vi "tvac_gui_chamber.vi"() -> ()   [LabVIEW 2016]
uses:
  <vilib>/httpClient/LabVIEWHTTPClient.lvlib
  <vilib>/httpClient/ClientHandle.ctl
  msg7171_linux.llb/send single message.vi
  <vilib>/httpClient/POSTBuffer.vi
panel:
  out "array w/ subset deleted":waveform(dbl)[](array[waveform])
  in  "AlarmColor":u32(colorbox)
  in  "Alarm String":string
  in  "Plot Color":u32(colorbox)=16860
  in  "Temperature":dbl format="%#_13g"
  in  "TC Label":string
  in  "Graph ON/OFF":u32(colorbox)=4250624
  in  "index (col)":i32
  in  "index (row)":i32
  out "working array":bool[](array[boolean])
  in  "Local Debug":bool
  in  "Tab Control":enum32{"TCs"}(tab)
  in  "Graphing Selection":u16(ring) items=["User Selection", "Graph All Thermocouples", "Clear Graph"]
  in  "Time Scale":u16(ring) items=["Minutes", "Hours", "Seconds"]
  out "Waveform Chart":waveform(dbl)[](graph)
  out "Thermocouples":T1(array[cluster])
  in  "exit":bool
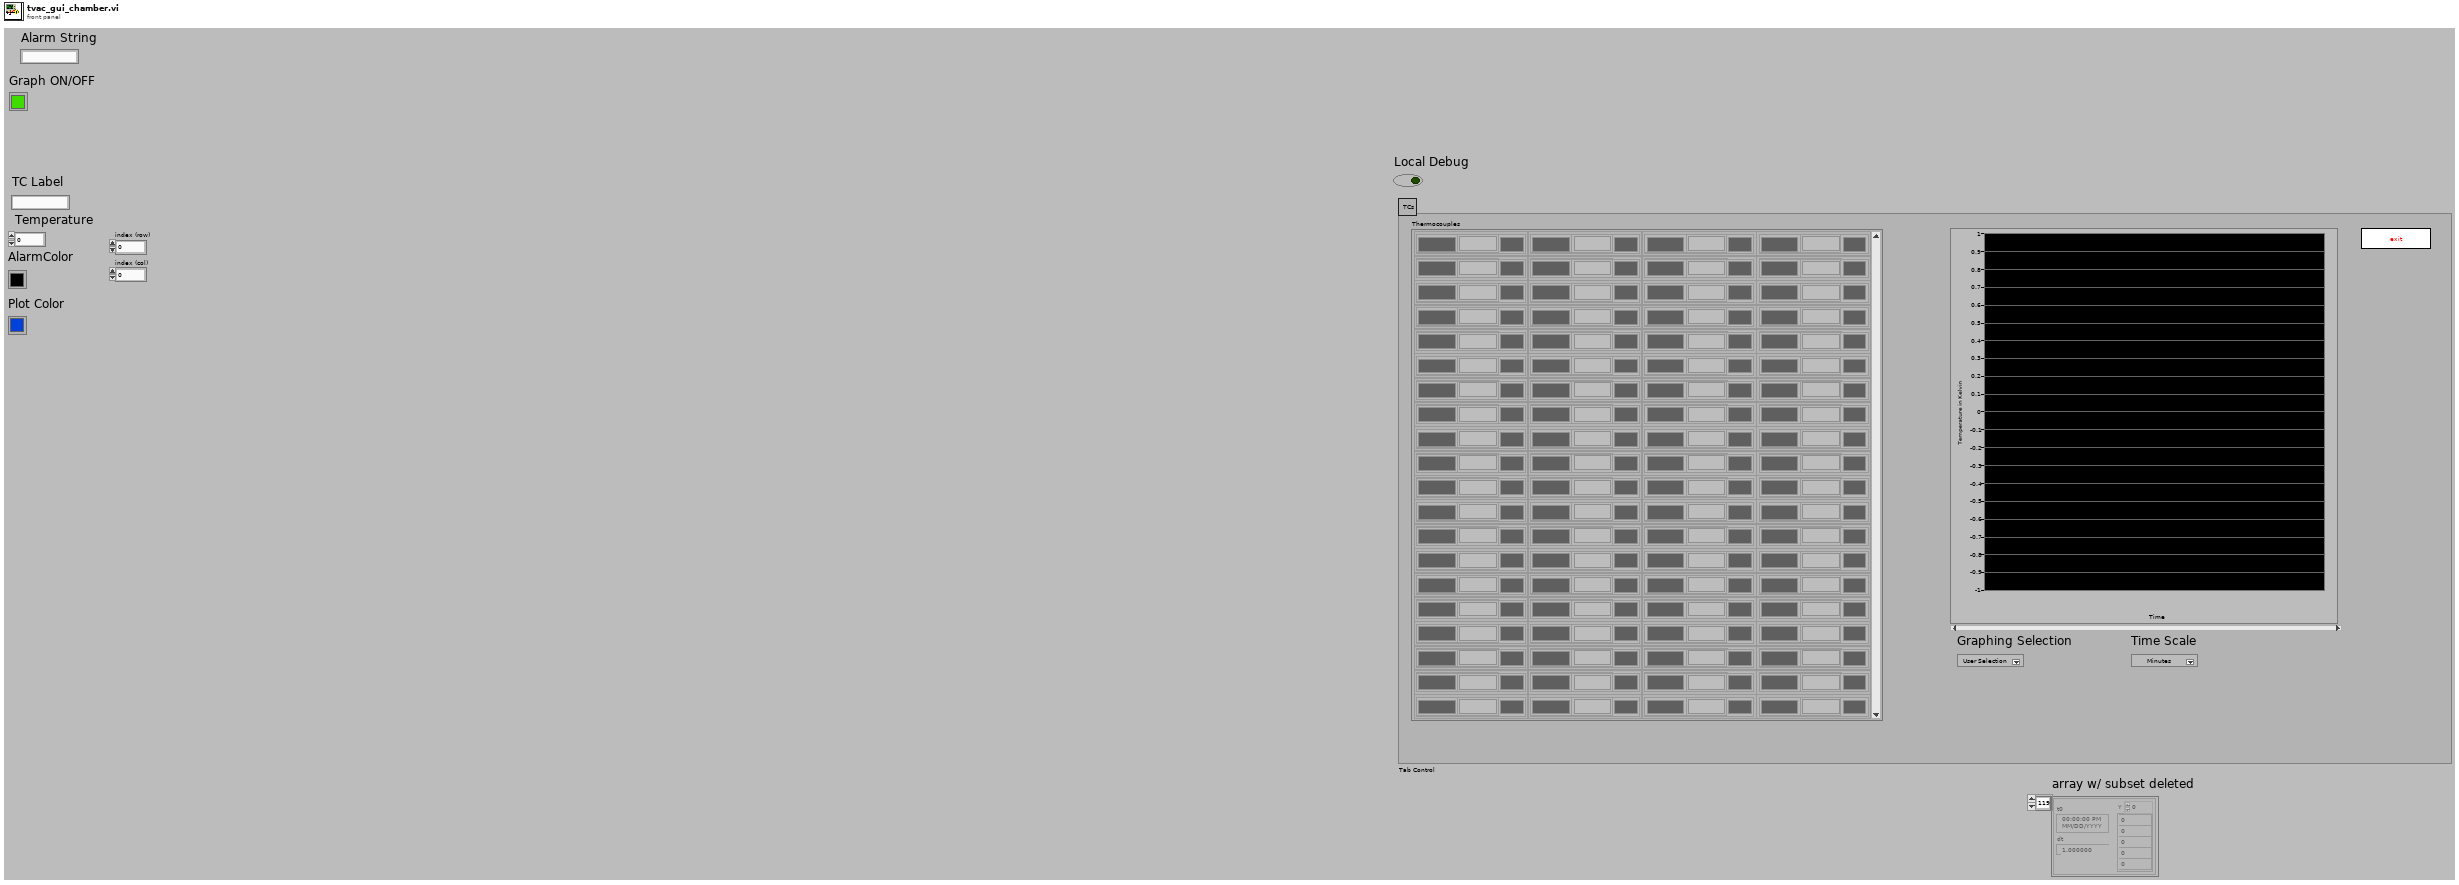
[diagram p1: front panel]
types:
  T1 = cluster{"TC Label":string, "Alarm Status":string, "Alarm Color":u32, "Temperature":string, "PlotColor":u32, "Graph On/Off":u32}[][]
  T2 = typedef "LabVIEWHTTPClient.lvlib/ClientHandle.ctl" = refnum<k1>
  T3 = cluster{"go":bool, "Http session":T2, "URL prefex":string, "index (row)":i32, "index (col)":i32, "Graph ON/OFF":u32, "TC Label":string, "Temperature":dbl, "AlarmColor":u32, "Plot Color":u32, "Alarm String":string, "Thermocouples":cluster{"TC Label":string, "Alarm Status":string, "Alarm Color":u32, "Temperature":string, "PlotColor":u32, "Graph On/Off":u32}[][], "working array":bool[], "i":i32, "NumberTCs":i32, "Waveform Chart":waveform(dbl)[]}
  T4 = cluster{"TC Label":string, "Alarm Status":string, "Alarm Color":u32, "Temperature":string, "PlotColor":u32, "Graph On/Off":u32}
  T5 = typedef "LVPoint32TypeDef.ctl" = cluster{"Horizontal":i32, "Vertical":i32}
  T6 = typedef "LVPositionTypeDef.ctl" = cluster{"Left":i32, "Top":i32}
  T7 = typedef "LVRangeTypeDef.ctl" = cluster{"Minimum":dbl, "Maximum":dbl, "Increment":dbl, "Minor Increment":dbl, "Start":dbl}
  T8 = cluster{"time":string, "TCs":cluster{"thermocouple":i32, "time":dbl, "temp":dbl, "working":bool, "alarm":i32}[]}
  T9 = cluster{"thermocouple":i32, "time":dbl, "temp":dbl, "working":bool, "alarm":i32}[]
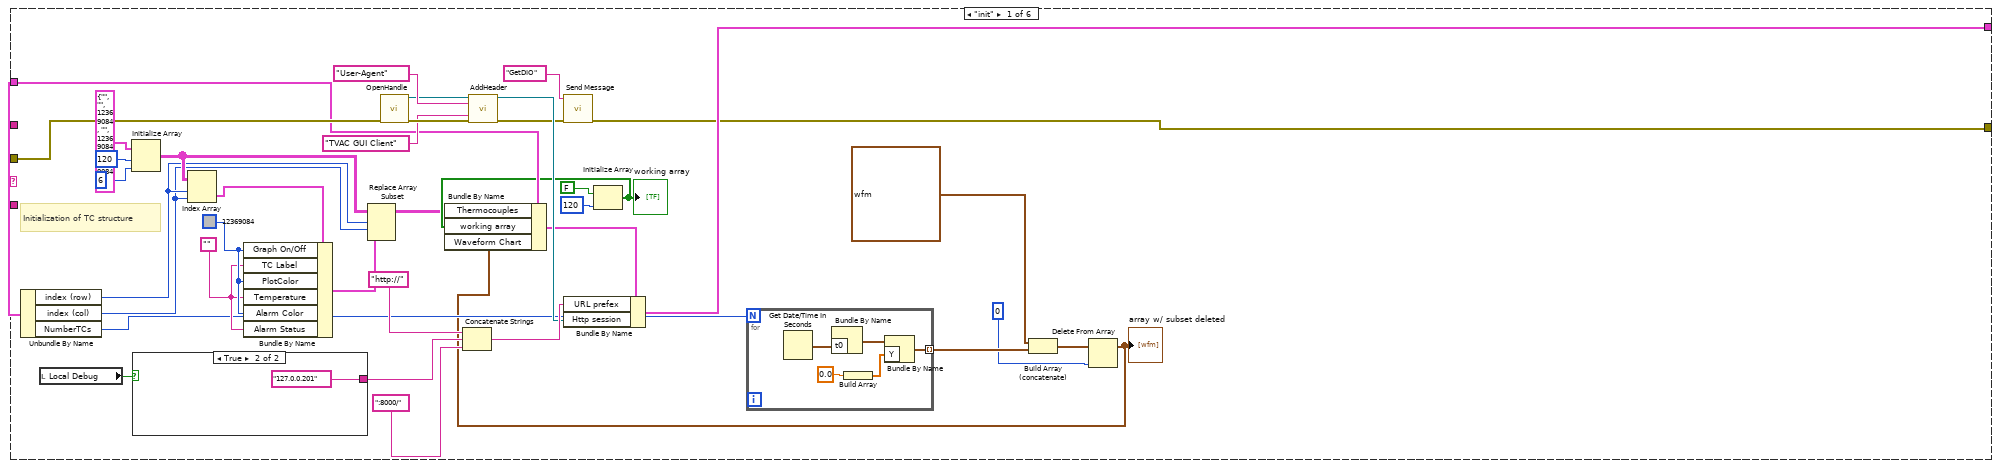
[diagram p2: hidden frame]
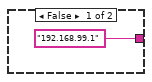
[diagram p3: hidden frame]
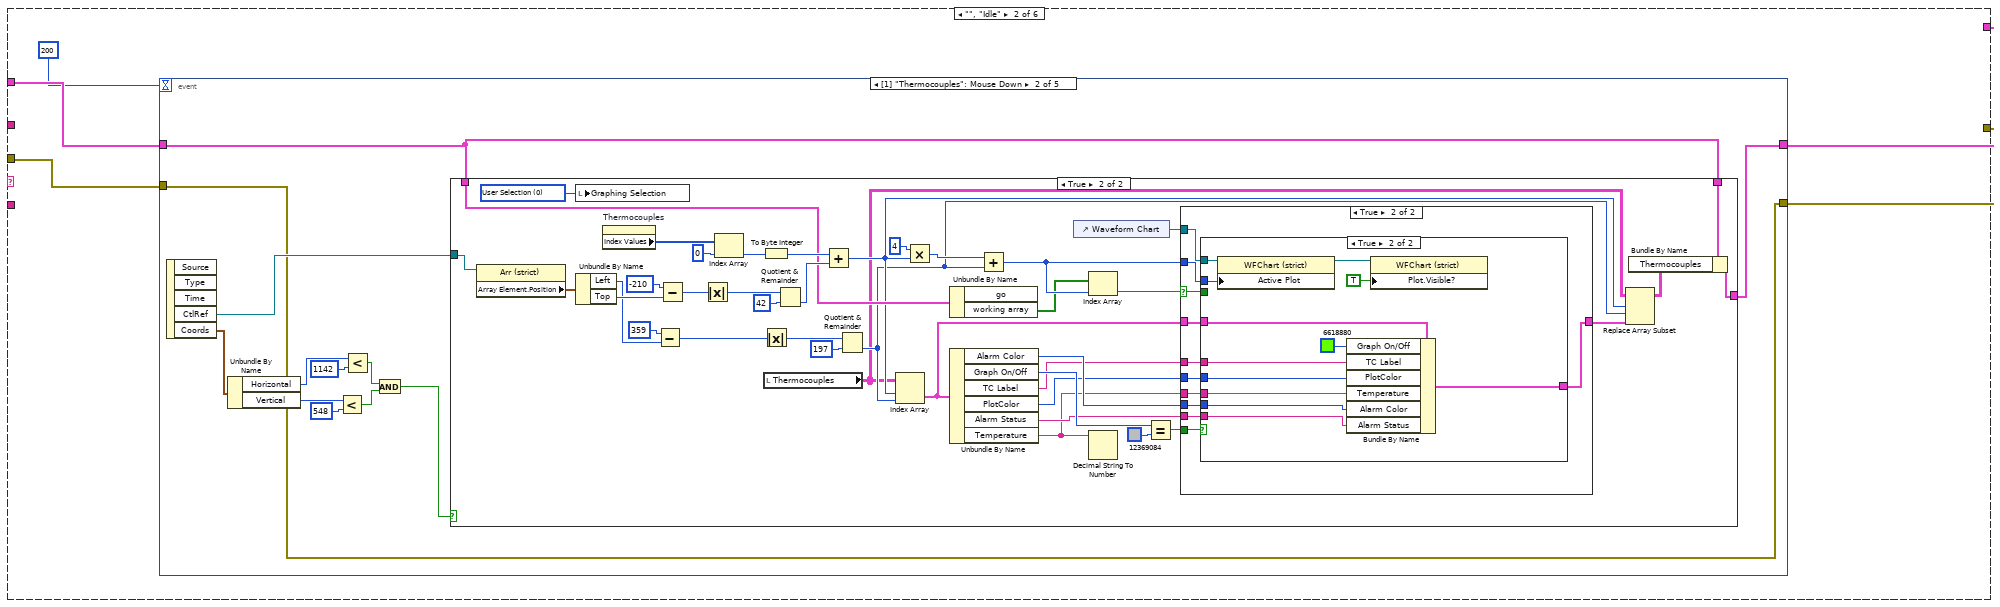
[diagram p4: hidden frame]
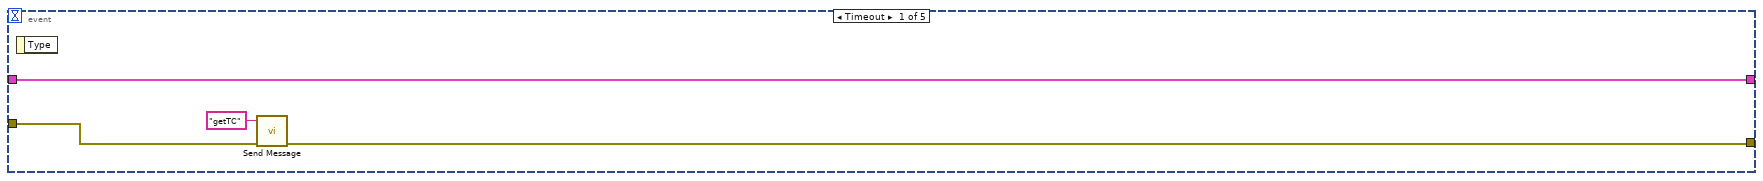
[diagram p5: hidden frame]
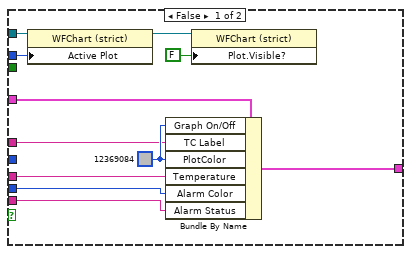
[diagram p8: hidden frame]
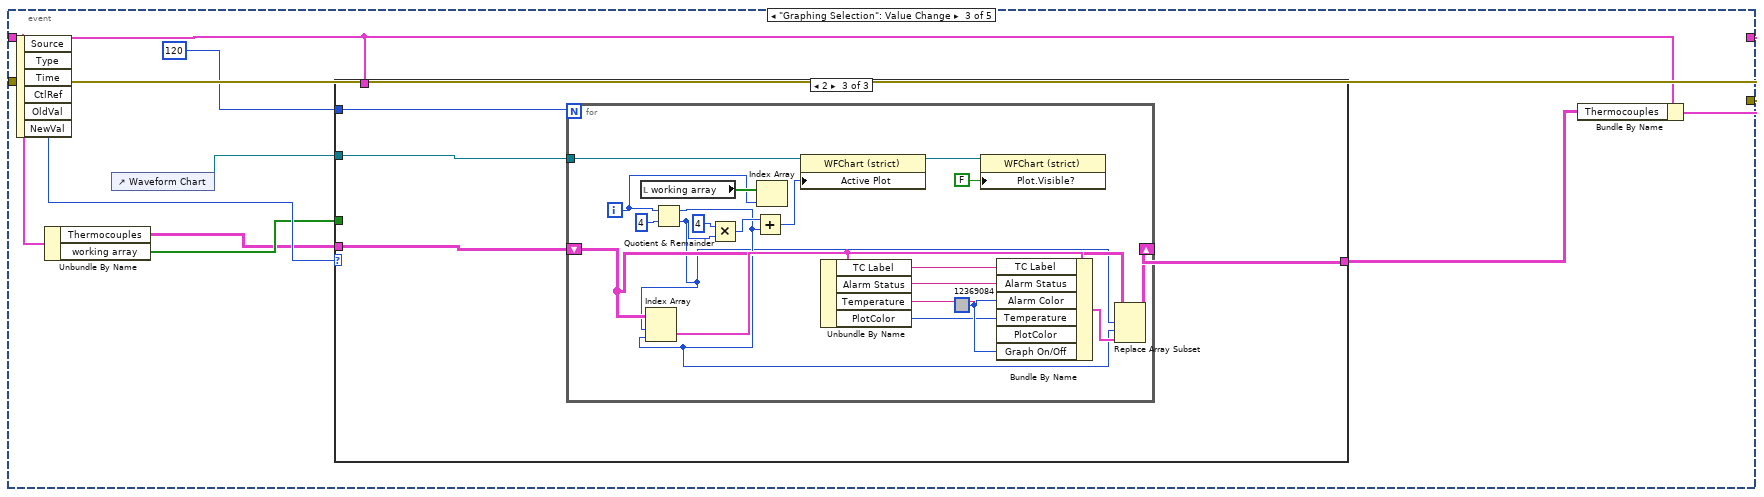
[diagram p9: hidden frame]
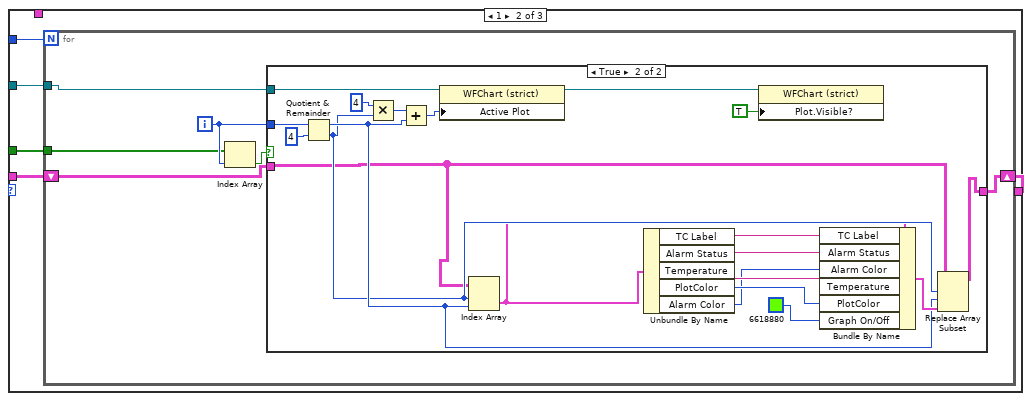
[diagram p11: hidden frame]
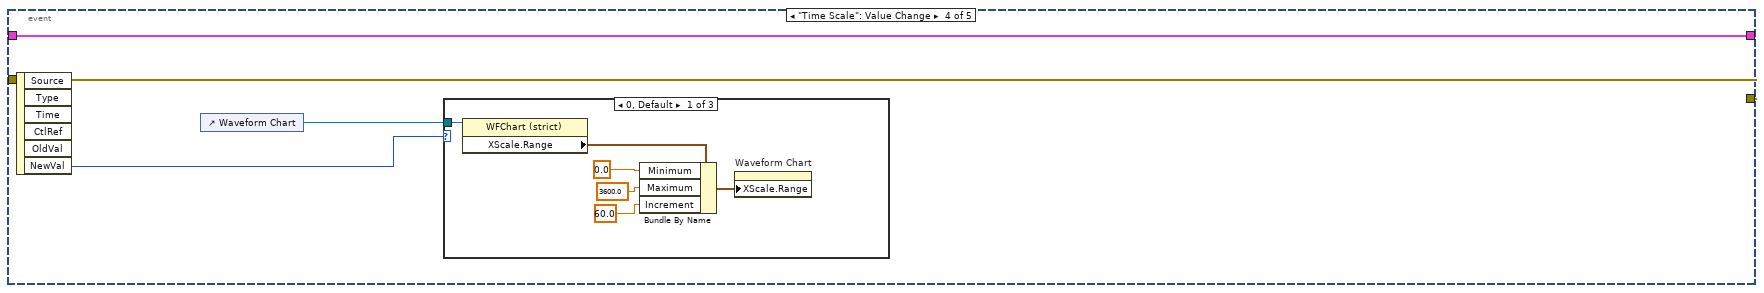
[diagram p13: hidden frame]
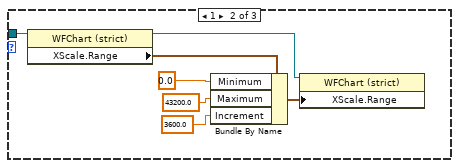
[diagram p14: hidden frame]
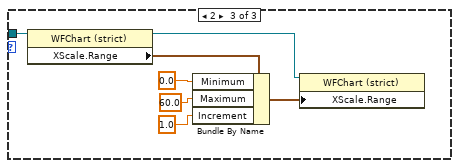
[diagram p15: hidden frame]
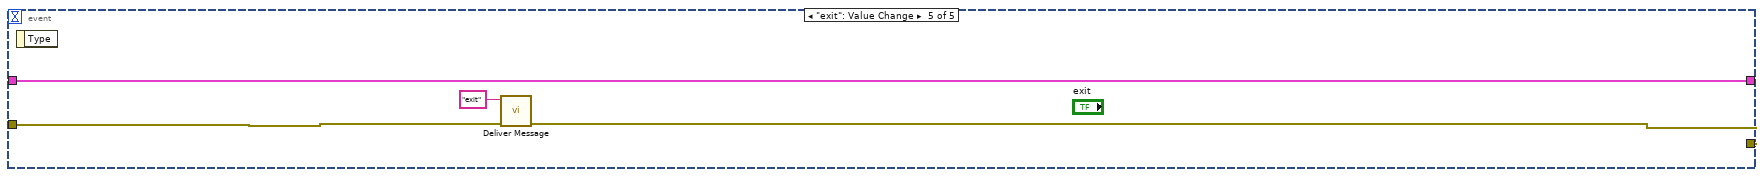
[diagram p16: hidden frame]
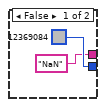
[diagram p17: hidden frame]
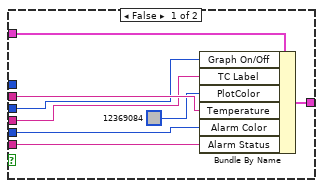
[diagram p18: hidden frame]
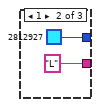
[diagram p19: hidden frame]
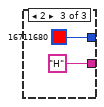
[diagram p20: hidden frame]
diagram:
  w19 = ""  # URL prefex
  w20 = T2 refnum  # Http session
  w21 = TRUE  # go
  n1 = call "Register Module.vi"() -> ("error out"=w17:errorcluster)  [unwired: 10 in, 1 out]
  n2 = call-poly "Send Message.vi"("error in (no error)"=w17, "event"="init") -> ("error out"=w16:errorcluster)  [unwired: 9 in]
  n3 = local read "Waveform Chart"() -> (w3:waveform(dbl)[])
  n4 = local read "Thermocouples"() -> (w2:T1)
  n5 = Bundle("go"=w21, "Http session"=w20, "URL prefex"=w19, "index (row)"="index (row)", "index (col)"="index (col)", "Graph ON/OFF"="Graph ON/OFF", "TC Label"="TC Label", "Temperature"="Temperature", "AlarmColor"="AlarmColor", "Plot Color"="Plot Color", "Alarm String"="Alarm String", "Thermocouples"=w2, "working array"=bool[] [TRUE, TRUE, TRUE, TRUE, TRUE, TRUE, TRUE, TRUE, TRUE, TRUE, TRUE, TRUE, TRUE, TRUE, TRUE, TRUE, TRUE, TRUE, TRUE, TRUE, TRUE, TRUE, TRUE, TRUE, TRUE, TRUE, TRUE, TRUE, TRUE, TRUE, TRUE, TRUE, TRUE, TRUE, TRUE, TRUE, TRUE, TRUE, TRUE, TRUE, TRUE, TRUE, TRUE, TRUE, TRUE, TRUE, TRUE, TRUE, TRUE, TRUE, TRUE, TRUE, TRUE, TRUE, TRUE, TRUE, TRUE, TRUE, TRUE, TRUE, TRUE, TRUE, TRUE, TRUE, TRUE, TRUE, TRUE, TRUE, TRUE, TRUE, TRUE, TRUE, TRUE, TRUE, TRUE, TRUE, TRUE, TRUE, TRUE, TRUE, TRUE, TRUE, TRUE, TRUE, TRUE, TRUE, TRUE, TRUE, TRUE, TRUE, TRUE, TRUE, TRUE, TRUE, TRUE, TRUE, TRUE, TRUE, TRUE, TRUE, TRUE, TRUE, TRUE, TRUE, TRUE, TRUE, TRUE, TRUE, TRUE, TRUE, TRUE, TRUE, TRUE, TRUE, TRUE, TRUE, TRUE, TRUE, TRUE, TRUE], "i"=0, "NumberTCs"=120, "Waveform Chart"=w3) -> (w7:T3)  [unwired: 1 in]
  n6 = while {
    shift-left: w7 -> [w26]
    shift-right: [w23] -> _
    shift-right: [w24] -> w1
    shift-left: w16 -> [w31]
    stop <- w22 continue-if-true
    n7 = call "Get Message.vi"("error in (no error)"=w31) -> ("error out"=w29:errorcluster, "event buffer"=w30:string, "event"=w28:string, "source"=w27:string)  [unwired: 7 in]
    n8 = case shown="\"getTC\"" w28 {
      selector: w28 -> [_ _ _ _ _ w432]
      tunnel: [w61 w78 w269 w401 w430 w434] -> w23
      tunnel: w26 -> [w41 w80 w275 w402 w425 w434]
      tunnel: w30 -> [_ _ _ _ _ _]
      tunnel: w29 -> [w64 w79 w296 w404 w428 w433]
      tunnel: [w57 w77 w270 w404 w427 w431] -> w25
      tunnel: w27 -> [_ _ _ _ _ _]
      frame "init" {
        w46 = ""
        w47 = u32 12369084 ("PlotColor")
        # "Initialization of TC structure"
        n9 = Unbundle By Name(w41) -> ("index (row)"=w49:i32, "index (col)"=w48:i32, "NumberTCs"=w38:i32)
        n10 = local read "Local Debug"() -> (w54:bool)
        n11 = Initialize Array(T4 {"TC Label"="", "Alarm Status"="", "Alarm Color"=12369084, "Temperature"="", "PlotColor"=12369084, "Graph On/Off"=12369084}, 120 ("dimension size"), 6 ("dimension size")) -> (w50:T1)
        n12 = case shown="True" w54 {
          tunnel: ["192.168.99.1" ("Address") "127.0.0.201" ("Address")] -> w55
          frame False {
          }
          frame True {
          }
        }
        n13 = Index Array(array=w50, index (row)=w49, index (col)=w48) -> (element=w45:T4)
        n14 = Bundle By Name(cluster=w45, "Graph On/Off"=w47, "TC Label"=w46, "PlotColor"=w47, "Temperature"=w46, "Alarm Color"=w47, "Alarm Status"=w46) -> (w44:T4)
        n15 = Replace Array Subset(array=w50, new element=w44, index (row)=w49, index (col)=w48) -> (w32:T1)
        n16 = call <vilib>:"OpenHandle.vi"("error in (no error)"=w64) -> ("client handle out"=w65:T2, "error out"=w68:errorcluster)  [unwired: 13 in]
        n17 = Concatenate Strings("http://" ("url"), w55, ":8000/" ("url")) -> (w60:string)
        n18 = call <vilib>:"AddHeader.vi"("client handle"=w65, "header"="User-Agent", "value"="TVAC GUI Client", "error in (no error)"=w68) -> ("client handle out"=w59:T2, "error out"=w58:errorcluster)  [unwired: 10 in]
        n19 = call-poly "Send Message.vi"("error in (no error)"=w58, "event"="GetDIO") -> ("error out"=w57:errorcluster)  [unwired: 9 in]
        n20 = Initialize Array(FALSE ("Boolean"), 120 ("dimension size")) -> (w39:bool[])
        "working array" <- w39
        n21 = for {
          N: w38 -> [_]
          tunnel: [w69] -> w36 mode=indexing
          n22 = Get Date/Time In Seconds() -> (seconds since 1Jan1904=w73:timestamp)
          n23 = Bundle By Name("t0"=w73) -> (w70:waveform(dbl))  [unwired: 1 in]
          n24 = Build Array(0.0) -> (w72:dbl[])
          n25 = Bundle By Name(cluster=w70, "Y"=w72) -> (w69:waveform(dbl))
        }
        n26 = Build Array (concatenate)(waveform(dbl) {"t0"=timestamp(0 s since 1904-01-01), "dt"=1.0, "Y"=[0.0]} ("element"), w36) -> (w37:waveform(dbl)[])
        n27 = Delete From Array(array=w37, index=0) -> (array with subset deleted=w35:waveform(dbl)[])  [unwired: 1 in, 1 out]
        "array w/ subset deleted" <- w35
        n28 = Bundle By Name(cluster=w41, "Thermocouples"=w32, "working array"=w39, "Waveform Chart"=w35) -> (w40:T3)
        n29 = Bundle By Name(cluster=w40, "URL prefex"=w60, "Http session"=w59) -> (w61:T3)
      }
      frame "", "Idle" {
        n30 = event shown="[1] \"Thermocouples\": Mouse Down" {
          selector: _ -> [_ _ _ _ _]
          dyn-events: _ -> [_ _ _ _ _]
          timeout: 200 ("milliseconds to wait") -> [_ _ _ _ _]
          tunnel: w79 -> [w82 w85 w180 w241 w266]
          tunnel: [w81 w85 w180 w241 w264] -> w77
          tunnel: [w84 w86 w175 w242 w267] -> w78
          tunnel: w80 -> [w84 w87 w176 w242 w267]
          event Timeout {
            n31 = event-data() -> ()  [unwired: 1 in, 1 out]
            n32 = call-poly "Send Message.vi"("error in (no error)"=w82, "event"="getTC") -> ("error out"=w81:errorcluster)  [unwired: 9 in]
          }
          event "Thermocouples": Mouse Down {
            n33 = event-data() -> ("CtlRef"=w89:refnum<vi>, "Coords"=w96:T5)  [unwired: 1 in, 3 out]
            n34 = Unbundle By Name(w96) -> ("Horizontal"=w94:i32, "Vertical"=w91:i32)
            n35 = Less?(x=w91, y=548) -> (x < y?=w90:bool)
            n36 = Less?(x=w94, y=1142) -> (x < y?=w95:bool)
            n37 = And(x=w95, y=w90) -> (x .and. y?=w88:bool)
            n38 = case shown="True" w88 {
              tunnel: w89 -> [_ w138]
              tunnel: w87 -> [_ w108]
              tunnel: w87 -> [w97 w106]
              tunnel: [w97 w98] -> w86
              frame False {
              }
              frame True {
                w132 = u16 0 items=["User Selection", "Graph All Thermocouples", "Clear Graph"] ("Graphing Selection")
                n39 = property class="Arr (strict)"(reference=w138) -> ("Array Element.Position"=w130:T6)  [unwired: 1 in, 2 out]
                n40 = local write "Graphing Selection"(w132) -> ()
                n41 = Unbundle By Name(w130) -> ("Left"=w127:i32, "Top"=w131:i32)
                n42 = property on="Thermocouples" class="Arr (strict)"() -> ("Index Values"=w121:u32[])  [unwired: 2 in, 2 out]
                n43 = Subtract(x=359, y=w127) -> (x-y=w126:i32)
                n44 = Subtract(x=-210, y=w131) -> (x-y=w118:i32)
                n45 = Absolute Value(x=w118) -> (abs(x)=w129:i32)
                n46 = Index Array(array=w121, index=0) -> (element=w117:u32)
                n47 = To Byte Integer(number=w117) -> (8bit integer=w116:i8)
                n48 = Absolute Value(x=w126) -> (abs(x)=w125:i32)
                n49 = local read "Thermocouples"() -> (w99:T1)
                n50 = Quotient & Remainder(x=w129, y=42) -> (floor(x/y)=w114:i32)  [unwired: 1 out]
                n51 = Add(x=w116, y=w114) -> (x+y=w101:i32)
                n52 = Quotient & Remainder(x=w125, y=197 ("Numeric 2")) -> (floor(x/y)=w100:i32)  [unwired: 1 out]
                n53 = Index Array(array=w99, index (row)=w101, index (col)=w100) -> (element=w102:T4)
                n54 = Multiply(x=4, y=w101) -> (x*y=w122:i32)
                n55 = Unbundle By Name(w108) -> ("working array"=w107:bool[])  [unwired: 1 out]
                n56 = Unbundle By Name(w102) -> ("Alarm Color"=w136:u32, "Graph On/Off"=w135:u32, "TC Label"=w134:string, "PlotColor"=w113:u32, "Alarm Status"=w133:string, "Temperature"=w104:string)
                n57 = Add(x=w122, y=w100) -> (x+y=w110:i32)
                n58 = control-ref of="Waveform Chart"() -> (w137:refnum<vi>)
                n59 = Index Array(array=w107, index=w110) -> (element=w109:bool)
                n60 = Decimal String To Number(string=w104) -> ()  [unwired: 2 in, 2 out]
                n61 = Equal?(x=w135, y=u32 12369084) -> (x = y?=w111:bool)
                n62 = case shown="True" w109 {
                  selector: w109 -> [_ w144]
                  tunnel: w137 -> [_ w150]
                  tunnel: w136 -> [_ w149]
                  tunnel: w134 -> [_ w148]
                  tunnel: w133 -> [_ w147]
                  tunnel: w110 -> [_ w140]
                  tunnel: w113 -> [_ w146]
                  tunnel: w111 -> [_ w145]
                  tunnel: w104 -> [_ w143]
                  tunnel: [w139 w142] -> w103
                  tunnel: w102 -> [w139 w141]
                  frame False {
                  }
                  frame True {
                    n63 = case shown="True" w145 {
                      tunnel: w150 -> [w160 w171]
                      tunnel: w149 -> [w154 w166]
                      tunnel: w148 -> [w155 w165]
                      tunnel: w147 -> [w156 w167]
                      tunnel: w146 -> [_ w169]
                      tunnel: w144 -> [_ _]
                      tunnel: w143 -> [w157 w168]
                      tunnel: [w152 w164] -> w142
                      tunnel: w141 -> [w153 w163]
                      tunnel: w140 -> [w151 w162]
                      frame False {
                        w158 = u32 12369084
                        n64 = property on="Property Node" class="WFChart (strict)"(reference=w160, "Active Plot"=w151) -> (reference out=w161:refnum<vi>)  [unwired: 1 in, 1 out]
                        n65 = Bundle By Name(cluster=w153, "Graph On/Off"=w158, "TC Label"=w155, "PlotColor"=w158, "Temperature"=w157, "Alarm Color"=w154, "Alarm Status"=w156) -> (w152:T4)
                        n66 = property class="WFChart (strict)"(reference=w161, "Plot.Visible?"=FALSE ("Plot.Visible")) -> ()  [unwired: 1 in, 2 out]
                      }
                      frame True {
                        n67 = property class="WFChart (strict)"(reference=w171, "Active Plot"=w162) -> (reference out=w172:refnum<vi>)  [unwired: 1 in, 1 out]
                        n68 = Bundle By Name(cluster=w163, "Graph On/Off"=u32 6618880, "TC Label"=w165, "PlotColor"=w169, "Temperature"=w168, "Alarm Color"=w166, "Alarm Status"=w167) -> (w164:T4)
                        n69 = property class="WFChart (strict)"(reference=w172, "Plot.Visible?"=TRUE ("Plot.Visible")) -> ()  [unwired: 1 in, 2 out]
                      }
                    }
                  }
                }
                n70 = Replace Array Subset(array=w99, new element=w103, index (row)=w101, index (col)=w100) -> (w105:T1)
                n71 = Bundle By Name(cluster=w106, "Thermocouples"=w105) -> (w98:T3)
              }
            }
          }
          event "Graphing Selection": Value Change {
            n72 = event-data() -> ("NewVal"=w181:u16)  [unwired: 1 in, 5 out]
            n73 = Unbundle By Name(w176) -> ("Thermocouples"=w174:T1, "working array"=w178:bool[])
            n74 = control-ref of="Waveform Chart"() -> (w182:refnum<vi>)
            n75 = case shown="2" w181 {
              tunnel: w174 -> [w183 w188 w219]
              tunnel: w182 -> [_ w187 w218]
              tunnel: 120 ("disabled index (col)") -> [_ w186 w217]
              tunnel: w176 -> [_ _ _]
              tunnel: w178 -> [_ w185 _]
              tunnel: [w183 w184 w216] -> w177
              frame 0, Default {
              }
              frame 1 {
                n76 = for {
                  N: w186 -> [_]
                  tunnel: w187 -> [w194]
                  shift-right: [w189] -> w184
                  shift-left: w188 -> [w193]
                  tunnel: w185 -> [w190]
                  i -> [w192]
                  n77 = Index Array(array=w190, index=w192) -> (element=w191:bool)
                  n78 = case shown="True" w191 {
                    tunnel: w194 -> [_ w215]
                    tunnel: w193 -> [w195 w196]
                    tunnel: [w195 w197] -> w189
                    tunnel: w192 -> [_ w214]
                    frame False {
                    }
                    frame True {
                      n79 = Quotient & Remainder(x=w214, y=4) -> (x-y*floor(x/y)=w200:i32, floor(x/y)=w199:i32)
                      n80 = Multiply(x=4, y=w199) -> (x*y=w210:i32)
                      n81 = Add(x=w210, y=w200) -> (x+y=w209:i32)
                      n82 = property class="WFChart (strict)"(reference=w215, "Active Plot"=w209) -> (reference out=w212:refnum<vi>)  [unwired: 1 in, 1 out]
                      n83 = Index Array(array=w196, index (row)=w199, index (col)=w200) -> (element=w198:T4)
                      n84 = Unbundle By Name(w198) -> ("TC Label"=w201:string, "Alarm Status"=w207:string, "Temperature"=w206:string, "PlotColor"=w203:u32, "Alarm Color"=w202:u32)
                      n85 = property class="WFChart (strict)"(reference=w212, "Plot.Visible?"=TRUE ("Plot.Visible")) -> ()  [unwired: 1 in, 2 out]
                      n86 = Bundle By Name(cluster=w198, "TC Label"=w201, "Alarm Status"=w207, "Alarm Color"=w202, "Temperature"=w206, "PlotColor"=w203, "Graph On/Off"=u32 6618880) -> (w205:T4)
                      n87 = Replace Array Subset(array=w196, new element=w205, index (row)=w199, index (col)=w200) -> (w197:T1)
                    }
                  }
                }
              }
              frame 2 {
                n88 = for {
                  N: w217 -> [_]
                  tunnel: w218 -> [w237]
                  shift-right: [w220] -> w216
                  shift-left: w219 -> [w224]
                  i -> [w238]
                  w230 = u32 12369084
                  n89 = local read "working array"() -> (w239:bool[])
                  n90 = Quotient & Remainder(x=w238, y=4 ("Numeric")) -> (x-y*floor(x/y)=w222:i32, floor(x/y)=w221:i32)
                  n91 = Index Array(array=w224, index (row)=w221, index (col)=w222) -> (element=w229:T4)
                  n92 = Multiply(x=4, y=w221) -> (x*y=w233:i32)
                  n93 = Add(x=w233, y=w222) -> (x+y=w232:i32)
                  n94 = Index Array(array=w239, index=w238) -> ()  [unwired: 1 out]
                  n95 = property class="WFChart (strict)"(reference=w237, "Active Plot"=w232) -> (reference out=w235:refnum<vi>)  [unwired: 1 in, 1 out]
                  n96 = Unbundle By Name(w229) -> ("TC Label"=w228:string, "Alarm Status"=w227:string, "Temperature"=w226:string, "PlotColor"=w225:u32)
                  n97 = property class="WFChart (strict)"(reference=w235, "Plot.Visible?"=FALSE ("Plot.Visible")) -> ()  [unwired: 1 in, 2 out]
                  n98 = Bundle By Name(cluster=w229, "TC Label"=w228, "Alarm Status"=w227, "Alarm Color"=w230, "Temperature"=w226, "PlotColor"=w225, "Graph On/Off"=w230) -> (w223:T4)
                  n99 = Replace Array Subset(array=w224, new element=w223, index (row)=w221, index (col)=w222) -> (w220:T1)
                }
              }
            }
            n100 = Bundle By Name(cluster=w176, "Thermocouples"=w177) -> (w175:T3)
          }
          event "Time Scale": Value Change {
            n101 = event-data() -> ("NewVal"=w243:u16)  [unwired: 1 in, 5 out]
            n102 = control-ref of="Waveform Chart"() -> (w240:refnum<vi>)
            n103 = case shown="0, Default" w243 {
              tunnel: w240 -> [w247 w251 w258]
              frame 0, Default {
                n104 = property on="Property Node" class="WFChart (strict)"(reference=w247) -> ("XScale.Range"=w249:T7)  [unwired: 1 in, 2 out]
                n105 = Bundle By Name(cluster=w249, "Minimum"=0.0, "Maximum"=3600.0, "Increment"=60.0) -> (w248:T7)
                n106 = property on="Waveform Chart" class="WFChart (strict)"("XScale.Range"=w248) -> ()  [unwired: 2 in, 2 out]
              }
              frame 1 {
                n107 = property on="Property Node" class="WFChart (strict)"(reference=w251) -> (reference out=w250:refnum<vi>, "XScale.Range"=w256:T7)  [unwired: 1 in, 1 out]
                n108 = Bundle By Name(cluster=w256, "Minimum"=0.0, "Maximum"=43200.0, "Increment"=3600.0) -> (w252:T7)
                n109 = property on="Property Node" class="WFChart (strict)"(reference=w250, "XScale.Range"=w252) -> ()  [unwired: 1 in, 2 out]
              }
              frame 2 {
                n110 = property on="Property Node" class="WFChart (strict)"(reference=w258) -> (reference out=w257:refnum<vi>, "XScale.Range"=w263:T7)  [unwired: 1 in, 1 out]
                n111 = Bundle By Name(cluster=w263, "Minimum"=0.0, "Maximum"=60.0, "Increment"=1.0) -> (w259:T7)
                n112 = property on="Property Node" class="WFChart (strict)"(reference=w257, "XScale.Range"=w259) -> ()  [unwired: 1 in, 2 out]
              }
            }
          }
          event "exit": Value Change {
            n113 = event-data() -> ()  [unwired: 1 in, 1 out]
            n114 = call "Deliver Message.vi"("error in (no error)"=w266, "event"="exit") -> ("error out"=w264:errorcluster)  [unwired: 9 in]
          }
        }
      }
      frame "getTC" {
        w287 = T8 {"time"="", "TCs"=[]} ("Cluster")
        n115 = property on="Waveform Chart" class="WFChart (strict)"("LegScrollVis"=TRUE ("Legend:Scrollbar Visible")) -> ()  [unwired: 2 in, 2 out]
        n116 = local read "Local Debug"() -> (w285:bool)
        n117 = Unbundle By Name(w275) -> ("Http session"=w294:T2, "URL prefex"=w292:string)
        n118 = Concatenate Strings(w292, "getAllThermoCoupleData" ("url")) -> (w293:string)
        n119 = Flatten To JSON(anything=w287) -> (JSON string=w286:string)  [unwired: 2 in, 1 out]
        n120 = case shown="True" w285 {
          tunnel: w296 -> [w370 w371]
          tunnel: [w369 w372] -> w271
          tunnel: [w368 w373] -> w295
          tunnel: w294 -> [w367 w376]
          tunnel: w293 -> [w366 w377]
          tunnel: [w365 w374] -> w290
          tunnel: [w364 w375] -> _
          tunnel: w286 -> [_ w378]
          frame False {
            n121 = call <vilib>:"GET.vi"("client handle"=w367, "url"=w366, "error in (no error)"=w370) -> ("client handle out"=w368:T2, "headers"=w364:string, "body"=w365:string, "error out"=w369:errorcluster)  [unwired: 9 in]
          }
          frame True {
            n122 = call-poly <vilib>:"POST.vi"("client handle"=w376, "url"=w377, "buffer"=w378, "error in (no error)"=w371) -> ("client handle out"=w373:T2, "headers"=w375:string, "body"=w374:string, "error out"=w372:errorcluster)  [unwired: 8 in]
          }
        }
        n123 = Bundle By Name(cluster=w275, "Http session"=w295) -> (w283:T3)
        n124 = call-poly "Send Message.vi"("error in (no error)"=w271, "event"="writeTC") -> ("error out"=w270:errorcluster)  [unwired: 9 in]
        n125 = Unflatten From JSON(JSON string=w290, type and defaults=w287) -> (value=w289:T8)  [unwired: 5 in, 1 out]
        n126 = Unbundle By Name(w283) -> ("working array"=w274:bool[], "Thermocouples"=w277:T1)  [unwired: 1 out]
        n127 = Unbundle By Name(w289) -> ("TCs"=w281:T9)
        n128 = for {
          N: 120 -> [_]
          tunnel: w281 -> [w325] mode=indexing
          tunnel: [w324] -> w268 mode=indexing
          shift-right: [w301] -> w276
          shift-left: w277 -> [w310]
          shift-right: [w300] -> w273
          shift-left: w274 -> [w299]
          i -> [w298]
          n129 = Quotient & Remainder(x=w298, y=4) -> (x-y*floor(x/y)=w308:i32, floor(x/y)=w309:i32)
          n130 = Unbundle By Name(w325) -> ("thermocouple"=w336:i32, "temp"=w297:dbl, "alarm"=w330:i32, "working"=w329:bool)
          n131 = Index Array(array=w310, index (row)=w309, index (col)=w308) -> (element=w321:T4)
          n132 = Index Array(array=w310, index (row)=w309, index (col)=w308) -> (element=w323:T4)
          n133 = Multiply(x=w309, y=4) -> (x*y=w331:i32)
          n134 = Multiply(x=w309, y=4) -> (x*y=w318:i32)
          n135 = Unbundle By Name(w323) -> ("Graph On/Off"=w307:u32)
          n136 = Add(x=w331, y=w308) -> (x+y=w326:i32)
          n137 = Add(x=w318, y=w308) -> (x+y=w316:i32)
          n138 = Replace Array Subset(array=w299, new element=w329, index=w298) -> (w300:bool[])
          n139 = To Double Precision Float(number=w297) -> (double precision float=w305:dbl)
          n140 = Get Date/Time In Seconds() -> (seconds since 1Jan1904=w328:timestamp)
          n141 = property on="Waveform Chart" class="WFChart (strict)"("Active Plot"=w326) -> ()  [unwired: 2 in, 2 out]
          n142 = Index Array(array=w300, index=w316) -> (element=w315:bool)
          n143 = Bundle By Name("t0"=w328) -> (w327:waveform(dbl))  [unwired: 1 in]
          n144 = Build Array(w305) -> (w334:dbl[])
          n145 = Number To Fractional String(number=w305, precision (6)=i16 2 ("width (-)")) -> (F-format string=w313:string)  [unwired: 2 in]
          n146 = case shown="True" w315 {
            tunnel: w307 -> [_ w341]
            tunnel: [u32 12369084 ("y") w341] -> w311
            tunnel: w313 -> [_ w340]
            tunnel: ["NaN" w340] -> w312
            frame False {
            }
            frame True {
            }
          }
          n147 = Bundle By Name(cluster=w327, "Y"=w334) -> (w324:waveform(dbl))
          n148 = Number To Decimal String(number=w336) -> (decimal integer string=w337:string)  [unwired: 1 in]
          n149 = case shown="0, Default" w330 {
            tunnel: ["" "L" "H"] -> w302
            tunnel: w330 -> [_ _ _]
            tunnel: [u32 12369084 u32 2812927 u32 16711680] -> w304
            frame 0, Default {
            }
            frame 1 {
            }
            frame 2 {
            }
          }
          n150 = property on="Waveform Chart" class="WFChart (strict)"() -> ("Plot.Plot Color"=w303:u32)  [unwired: 2 in, 2 out]
          n151 = Concatenate Strings("TC " ("string"), w337) -> (w306:string)
          n152 = Equal?(x=w311, y=u32 6618880) -> (x = y?=w319:bool)
          n153 = case shown="True" w319 {
            tunnel: [w349 w357] -> w322
            tunnel: w321 -> [w348 w356]
            tunnel: w311 -> [w346 w355]
            tunnel: w312 -> [w347 w354]
            tunnel: w306 -> [w345 w353]
            tunnel: w304 -> [w344 w352]
            tunnel: w303 -> [_ w351]
            tunnel: w302 -> [w343 w350]
            frame False {
              n154 = Bundle By Name(cluster=w348, "Graph On/Off"=w346, "TC Label"=w345, "PlotColor"=u32 12369084 ("y"), "Temperature"=w347, "Alarm Color"=w344, "Alarm Status"=w343) -> (w349:T4)
            }
            frame True {
              n155 = Bundle By Name(cluster=w356, "Graph On/Off"=w355, "TC Label"=w353, "PlotColor"=w351, "Temperature"=w354, "Alarm Color"=w352, "Alarm Status"=w350) -> (w357:T4)
            }
          }
          n156 = property on="Waveform Chart" class="WFChart (strict)"("Plot.Plot Name"=w306) -> ()  [unwired: 2 in, 2 out]
          n157 = Replace Array Subset(array=w310, new element=w322, index (row)=w309, index (col)=w308) -> (w301:T1)
        }
        n158 = Bundle By Name(cluster=w275, "Thermocouples"=w276, "working array"=w273) -> (w269:T3)
        n159 = Build Array (concatenate)(waveform(dbl) {"t0"=timestamp(0 s since 1904-01-01), "dt"=1.0, "Y"=[]} ("element"), w268) -> (w280:waveform(dbl)[])
        n160 = local write "Thermocouples"(w276) -> ()
        n161 = Delete From Array(array=w280, index=0) -> (array with subset deleted=→"Waveform Chart":waveform(dbl)[])  [unwired: 1 in, 1 out]
      }
      frame "writeTC" {
        n162 = Unbundle By Name(w402) -> ("Thermocouples"=w403:T1, "index (row)"=w394:i32, "index (col)"=w393:i32, "Graph ON/OFF"=w389:u32, "TC Label"=w384:string, "Temperature"=w387:dbl, "AlarmColor"=w383:u32, "Plot Color"=w382:u32, "Alarm String"=w381:string, "working array"=w391:bool[])
        n163 = Index Array(array=w403, index (row)=w394, index (col)=w393) -> (element=w399:T4)
        n164 = Multiply(x=w394, y=4) -> (x*y=w396:i32)
        n165 = Add(x=w396, y=w393) -> (x+y=w392:i32)
        n166 = Index Array(array=w391, index=w392) -> (element=w390:bool)
        n167 = Number To Fractional String(number=w387, precision (6)=i16 2 ("width (-)")) -> (F-format string=w386:string)  [unwired: 2 in]
        n168 = case shown="True" w390 {
          tunnel: w389 -> [_ w408]
          tunnel: [u32 12369084 ("y") w408] -> w380
          tunnel: w386 -> [_ w407]
          tunnel: ["NaN" w407] -> w385
          frame False {
          }
          frame True {
          }
        }
        n169 = Equal?(x=w380, y=u32 6618880) -> (x = y?=w397:bool)
        n170 = case shown="False" w397 {
          tunnel: [w416 w424] -> w400
          tunnel: w399 -> [w415 w423]
          tunnel: w380 -> [w413 w422]
          tunnel: w385 -> [w414 w421]
          tunnel: w384 -> [w412 w420]
          tunnel: w383 -> [w411 w419]
          tunnel: w382 -> [_ w418]
          tunnel: w381 -> [w410 w417]
          frame False {
            n171 = Bundle By Name(cluster=w415, "Graph On/Off"=w413, "TC Label"=w412, "PlotColor"=u32 12369084 ("y"), "Temperature"=w414, "Alarm Color"=w411, "Alarm Status"=w410) -> (w416:T4)
          }
          frame True {
            n172 = Bundle By Name(cluster=w423, "Graph On/Off"=w422, "TC Label"=w420, "PlotColor"=w418, "Temperature"=w421, "Alarm Color"=w419, "Alarm Status"=w417) -> (w424:T4)
          }
        }
        n173 = Replace Array Subset(array=w403, new element=w400, index (row)=w394, index (col)=w393) -> (w379:T1)
        n174 = Bundle By Name(cluster=w402, "Thermocouples"=w379) -> (w401:T3)
        n175 = local write "Thermocouples"(w379) -> ()
      }
      frame "exit" {
        n176 = Unbundle By Name(w425) -> ("Http session"=w426:T2)
        n177 = call <vilib>:"CloseHandle.vi"("client handle"=w426, "error in (no error)"=w428) -> ("error out"=w427:errorcluster)  [unwired: 13 in]
        n178 = Bundle By Name(cluster=w425, "go"=FALSE ("Bundle Element")) -> (w430:T3)
      }
      frame Default {
        n179 = call "Unknown Message Dialog.vi"("error in (no error)"=w433, "event name"=w432) -> ("error out"=w431:errorcluster)  [unwired: 9 in]
      }
    }
    n180 = Unbundle By Name(w23) -> ("go"=w22:bool)
    n181 = call "log system event.vi"("error in (no error)"=w25) -> ("error out"=w24:errorcluster)  [unwired: 9 in, 1 out]
  }
  n182 = call "Unload Module.vi"("error in (no error)"=w1) -> ()  [unwired: 10 in, 1 out]
  n183 = property on="Waveform Chart" class="WFChart (strict)" props=["Plot", "Visible?"]() -> ()  [unwired: 2 in, 3 out]
